vi "b-field one sensor tx ty.vi"(0 "magnet location params":T1, 7 "x sensor":dbl, 9 "y sensor":dbl, 11 "z sensor":dbl) -> (4 "Bx,By,Bz (uT)":dbl[](array[numeric]), 6 "dB (x,y,z, tx, ty, BrV)":dbl[][](array[numeric]))   [LabVIEW 2017]
uses:
  typedefs/magnet location tx ty.ctl
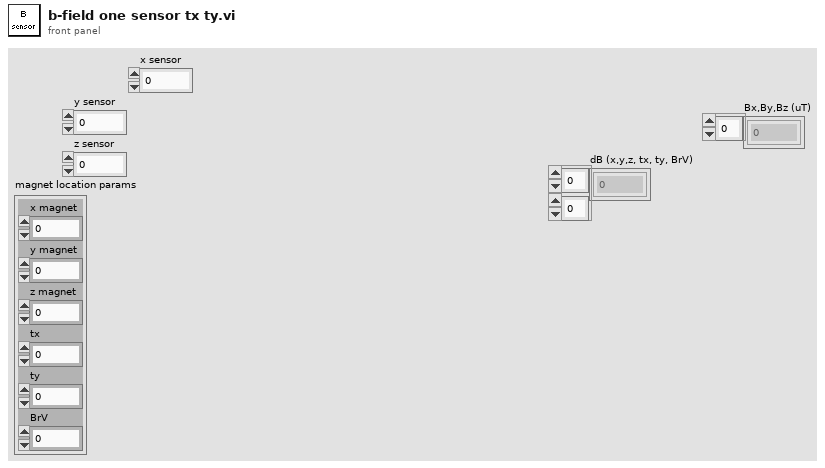
[diagram p1: front panel]
types:
  T1 = typedef "magnet location tx ty.ctl" = cluster{"x magnet":dbl, "y magnet":dbl, "z magnet":dbl, "tx":dbl, "ty":dbl, "BrV":dbl}
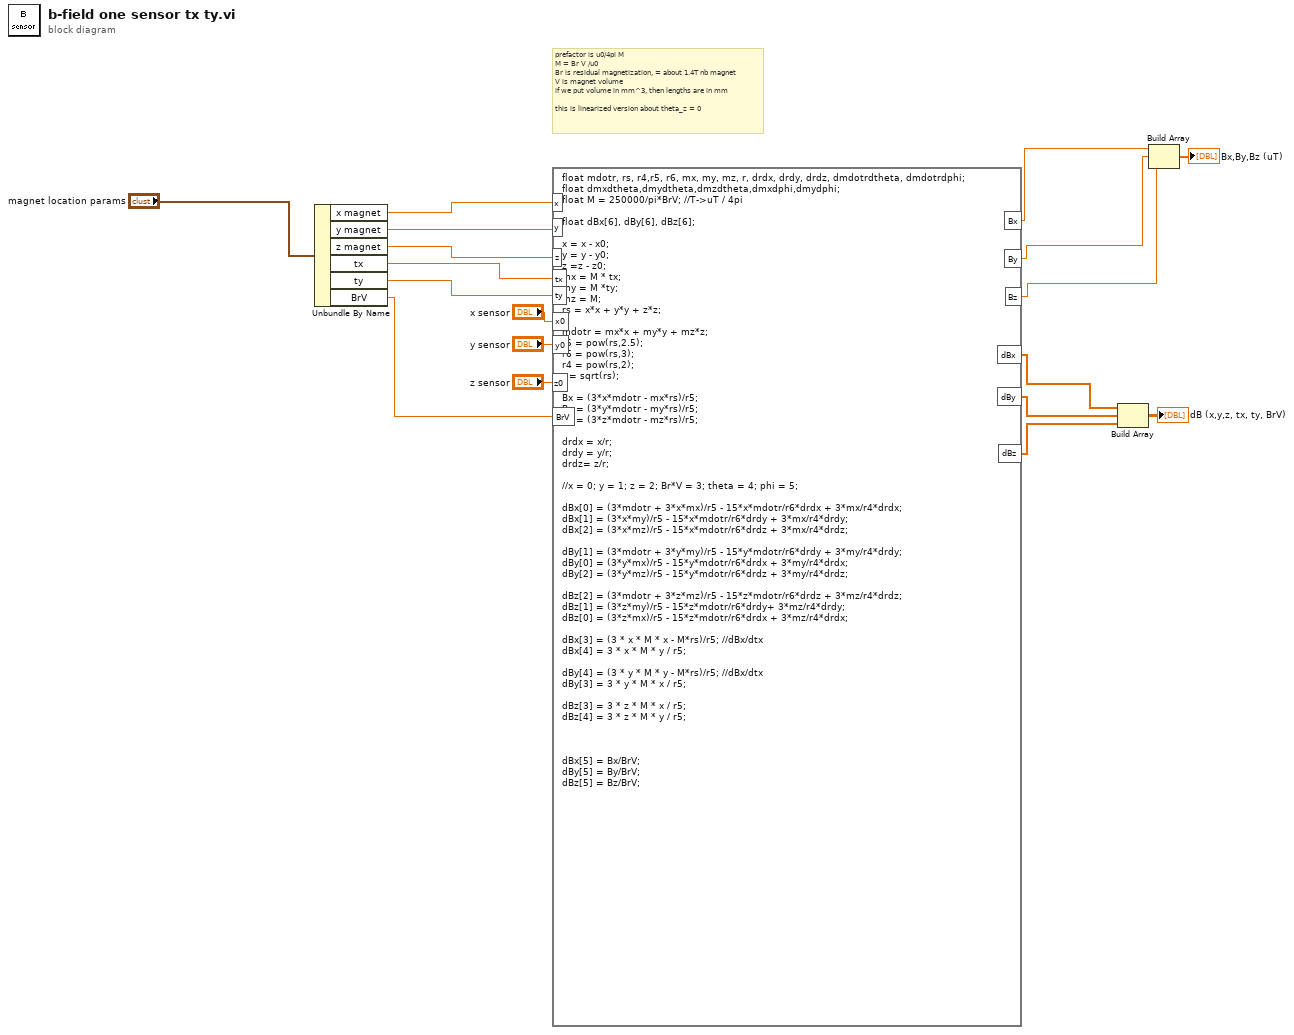
[diagram p0: block diagram]
diagram:
  # "prefactor is u0/4pi M\nM = Br V /u0\nBr is residual magnetization, = about 1.4T nb magnet\nV is magnet volume\nif we put volume in mm^3, then lengths are in mm\n\nthis is linearized version about theta_z = 0"
  n1 = Unbundle By Name("magnet location params") -> ("x magnet"=w14:dbl, "y magnet"=w13:dbl, "z magnet"=w12:dbl, "tx"=w11:dbl, "ty"=w10:dbl, "BrV"=w1:dbl)
  n2 = formula code="float mdotr, rs, r4,r5, r6, mx, my, mz, r, drdx, drdy, drdz, dmdotrdtheta, dmdotrdphi;\nfloat dmxdtheta,dmydtheta,dmzdtheta,dmxdphi,dmydphi;\nfloat M = 250000/pi*BrV; //T->uT / 4pi\n\nfloat dBx[6], dBy[6], dBz[6];\n\nx = x - x0;\ny = y - y0;\nz =z - z0;\nmx = M * tx;\nmy = M *ty;\nmz = M;\nrs = x*x + y*y + z*z;\n\nmdotr = mx*x + my*y + mz*z;\nr5 = pow(rs,2.5);\nr6 = pow(rs,3);\nr4 = pow(rs,2);\nr = sqrt(rs);\n\nBx = (3*x*mdotr - mx*rs)/r5;\nBy = (3*y*mdotr - my*rs)/r5;\nBz = (3*z*mdotr - mz*rs)/r5;\n\ndrdx = x/r;\ndrdy = y/r;\ndrdz= z/r;\n\n//x = 0; y = 1; z = 2; Br*V = 3; theta = 4; phi = 5;\n\ndBx[0] = (3*mdotr + 3*x*mx)/r5 - 15*x*mdotr/r6*drdx + 3*mx/r4*drdx;\ndBx[1] = (3*x*my)/r5 - 15*x*mdotr/r6*drdy + 3*mx/r4*drdy;\ndBx[2] = (3*x*mz)/r5 - 15*x*mdotr/r6*drdz + 3*mx/r4*drdz;\n\ndBy[1] = (3*mdotr + 3*y*my)/r5 - 15*y*mdotr/r6*drdy + 3*my/r4*drdy;\ndBy[0] = (3*y*mx)/r5 - 15*y*mdotr/r6*drdx + 3*my/r4*drdx;\ndBy[2] = (3*y*mz)/r5 - 15*y*mdotr/r6*drdz + 3*my/r4*drdz;\n\ndBz[2] = (3*mdotr + 3*z*mz)/r5 - 15*z*mdotr/r6*drdz + 3*mz/r4*drdz;\ndBz[1] = (3*z*my)/r5 - 15*z*mdotr/r6*drdy+ 3*mz/r4*drdy;\ndBz[0] = (3*z*mx)/r5 - 15*z*mdotr/r6*drdx + 3*mz/r4*drdx;\n\ndBx[3] = (3 * x * M * x - M*rs)/r5; //dBx/dtx\ndBx[4] = 3 * x * M * y / r5;\n\ndBy[4] = (3 * y * M * y - M*rs)/r5; //dBx/dtx\ndBy[3] = 3 * y * M * x / r5;\n\ndBz[3] = 3 * z * M * x / r5;\ndBz[4] = 3 * z * M * y / r5;\n\n\n\ndBx[5] = Bx/BrV;\ndBy[5] = By/BrV;\ndBz[5] = Bz/BrV;"("x"=w14, "y"=w13, "z"=w12, "x0"="x sensor", "y0"="y sensor", "z0"="z sensor", "BrV"=w1, "tx"=w11, "ty"=w10) -> ("Bx"=w9:dbl, "By"=w8:dbl, "Bz"=w7:dbl, "dBx"=w5:dbl[], "dBy"=w4:dbl[], "dBz"=w3:dbl[])
  n3 = Build Array(w5, w4, w3) -> (→"dB (x,y,z, tx, ty, BrV)":dbl[][])
  n4 = Build Array(w9, w8, w7) -> (→"Bx,By,Bz (uT)":dbl[])
